vi "Set.vi"(0 "reference in":refnum<class "Mediator.lvclass">, 2 "Colleague":refnum<class "Colleague.lvclass">[](array[class]), 5 "error in (no error)":errorcluster) -> (14 "reference out":refnum<class "Mediator.lvclass">, 19 "error out":errorcluster)   [LabVIEW 2013, in "Mediator.lvclass"]
uses:
  Mediator.lvclass
  Colleague_class/Colleague.lvclass
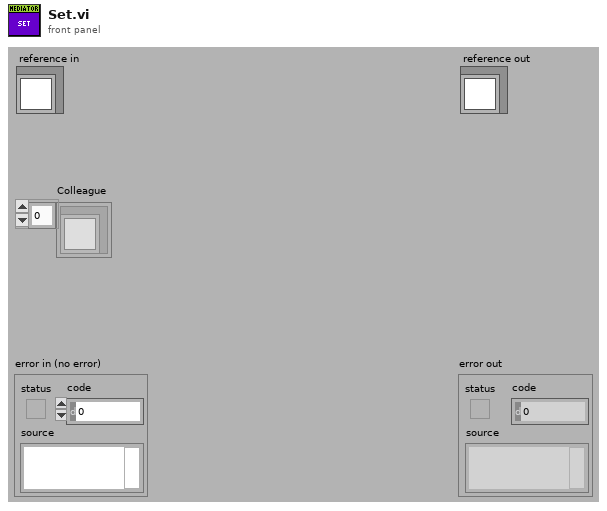
[diagram p1: front panel]
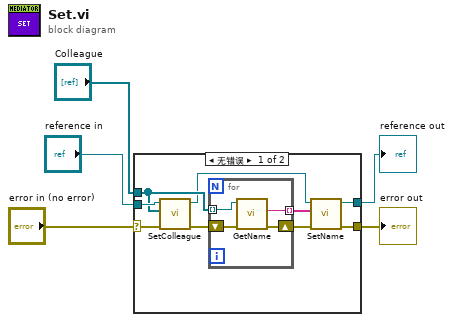
[diagram p0: block diagram]
diagram:
  n1 = case shown="无错误" "error in (no error)" {
    selector: "error in (no error)" -> [w7 w20]
    tunnel: [w6 w20] -> w4
    tunnel: [w8 w19] -> w2
    tunnel: "reference in" -> [w14 w19]
    tunnel: "Colleague" -> [w13 _]
    frame No Error {
      n2 = call-dynamic "SetColleague.vi"("error in (no error)"=w7, "Colleague"=w13, "reference in"=w14) -> ("error out"=w11:errorcluster, "reference out"=w10:refnum<class "Mediator.lvclass">)  [unwired: 7 in]
      n3 = for {
        tunnel: w13 -> [w18] mode=indexing
        tunnel: [w17] -> w12 mode=indexing
        shift-right: [w15] -> w9
        shift-left: w11 -> [w16]
        n4 = call "GetName.vi"("error in (no error)"=w16, "reference in"=w18) -> ("error out"=w15:errorcluster, "Name"=w17:string)  [unwired: 7 in, 1 out]
      }
      n5 = call-dynamic "SetName.vi"("error in (no error)"=w9, "Name"=w12, "reference in"=w10) -> ("error out"=w6:errorcluster, "reference out"=w8:refnum<class "Mediator.lvclass">)  [unwired: 7 in]
    }
    frame Error {
    }
  }
  "error out" <- w4
  "reference out" <- w2
